vi "Prober_ValidCoordinate.vi"(8 "error in (no error)":errorcluster, 9 "Axis":enum16{"X", "Y", "Z", "Theta"}(ring), 10 "Coordinate IN":i32, 11 "SemiProbe in":refnum<class "SemiProbe.lvclass">) -> (0 "error out":errorcluster, 2 "Is Valid?":bool, 3 "SemiProbe out":refnum<class "SemiProbe.lvclass">)   [LabVIEW 2019, in "SemiProbe.lvclass"]
uses:
  SemiProbe.lvclass
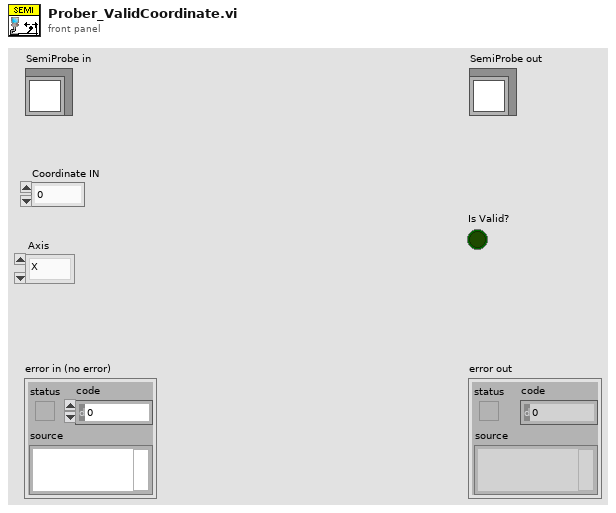
[diagram p1: front panel]
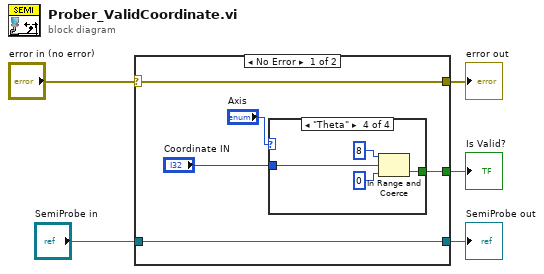
[diagram p0: block diagram]
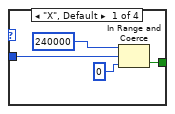
[diagram p2: hidden frame]
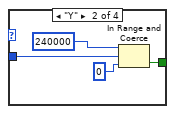
[diagram p3: hidden frame]
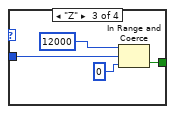
[diagram p4: hidden frame]
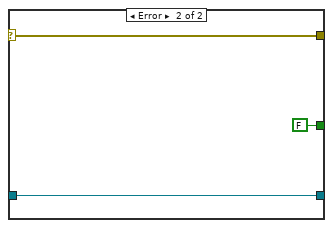
[diagram p5: hidden frame]
diagram:
  n1 = case shown="No Error" "error in (no error)" {
    selector: "error in (no error)" -> [w7 w27]
    tunnel: [w8 FALSE] -> w4
    tunnel: [w7 w27] -> w3
    tunnel: "SemiProbe in" -> [w6 w28]
    tunnel: [w6 w28] -> w1
    frame No Error {
      n2 = case shown="\"Theta\"" "Axis" {
        tunnel: "Coordinate IN" -> [w13 w16 w20 w24]
        tunnel: [w11 w15 w19 w23] -> w8
        frame "X", Default {
          n3 = In Range and Coerce(upper limit=240000, x=w13, lower limit=0) -> (In Range?=w11:bool)  [unwired: 1 out]
        }
        frame "Y" {
          n4 = In Range and Coerce(upper limit=240000, x=w16, lower limit=0) -> (In Range?=w15:bool)  [unwired: 1 out]
        }
        frame "Z" {
          n5 = In Range and Coerce(upper limit=12000, x=w20, lower limit=0) -> (In Range?=w19:bool)  [unwired: 1 out]
        }
        frame "Theta" {
          n6 = In Range and Coerce(upper limit=8, x=w24, lower limit=0) -> (In Range?=w23:bool)  [unwired: 1 out]
        }
      }
    }
    frame Error {
    }
  }
  "error out" <- w3
  "SemiProbe out" <- w1
  "Is Valid?" <- w4
